vi "FTW-Actor-Initialize.vi"(0 "Uninitialized FTW Actor":refnum<class "FTW-Actor.lvclass">, 5 "Actor Ref Prototype":refnum<class "FTW-ActorReference.lvclass">, 7 "Initialization Job Sequence":string, 11 "error in":errorcluster) -> (4 "FTW Actor":refnum<class "FTW-Actor.lvclass">, 15 "error out":errorcluster)   [LabVIEW 2015, in "FTW-Actor.lvclass"]
uses:
  FTW-Actor.lvclass
  Reference/FTW-ActorReference.lvclass
  Sequencer/FTW-Sequencer.lvclass/FTW-Sequencer.ctl
  FTW-Actor.lvclass/FTW-Actor.ctl
  Sequencer/FTW-Sequencer.lvclass
panel:
  # "Inputs"
  # "Outputs"
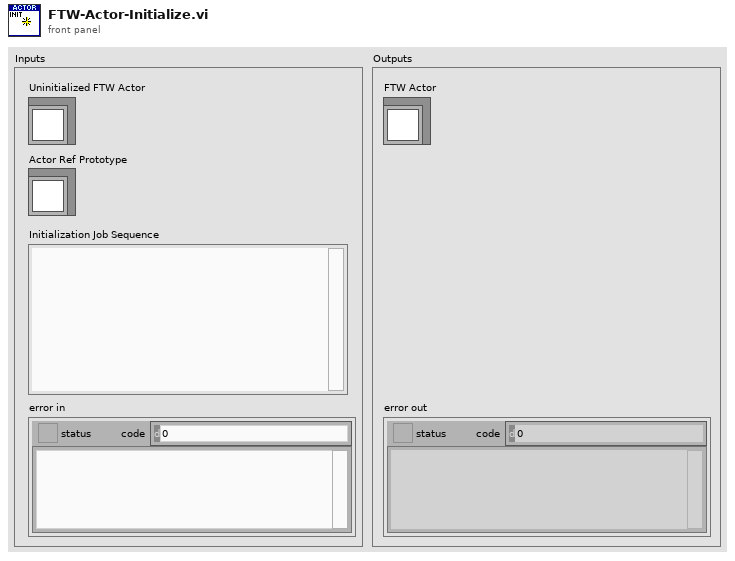
[diagram p1: front panel]
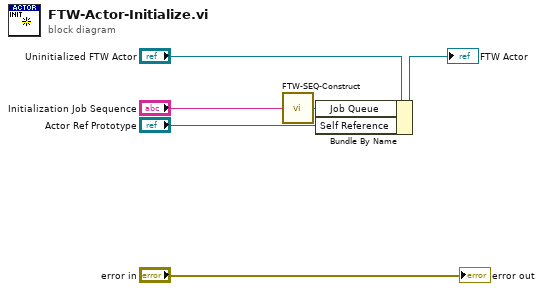
[diagram p0: block diagram]
diagram:
  n1 = call "FTW-SEQ-Construct.vi"("Initial Sequence"="Initialization Job Sequence") -> ("Sequencer"=w5:refnum<class "FTW-Sequencer.lvclass">)
  n2 = Bundle By Name(cluster="Uninitialized FTW Actor", "Job Queue"=w5, "Self Reference"="Actor Ref Prototype") -> (→"FTW Actor":refnum<class "FTW-Actor.lvclass">)
  "error out" <- "error in"
